vi "FunctionalTest.vi"() -> ()   [LabVIEW 2018]
panel:
  out "TEST RESULT":bool
  out "Functional Test\nErrors":bool[](array[boolean])
  out "SAT":u32[](array[numeric])
  out "HUE":dbl[](array[numeric])
  in  "Port selection":refnum<visa-resource-name>="ASRL27::INSTR"
  out "Status":string
  out "LED 20":bool
  out "LED 19":bool
  out "LED 18":bool
  out "LED 17":bool
  out "LED 16":bool
  out "LED 15":bool
  out "LED 14":bool
  out "LED 13":bool
  out "LED 12":bool
  out "LED 11":bool
  out "LED 10":bool
  out "LED 9":bool
  out "LED 8":bool
  out "LED 7":bool
  out "LED 6":bool
  out "LED 5":bool
  out "LED 4":bool
  out "LED 3":bool
  out "LED 2":bool
  out "LED":bool
  out "INTENSITY":u32[](array[numeric])
  out "BLUE":u8[](array[numeric])
  out "GREEN":u8[](array[numeric])
  out "RED":u8[](array[numeric])
  in  "CAPTURE\n& READ":bool
  in  "stop":bool
  # "Fiber"
  # "1"
  # "2"
  # "3"
  # "4"
  # "5"
  # "6"
  # "7"
  # "8"
  # "9"
  # "10"
  # "11"
  # "12"
  # "13"
  # "14"
  # "15"
  # "16"
  # "17"
  # "18"
  # "19"
  # "20"
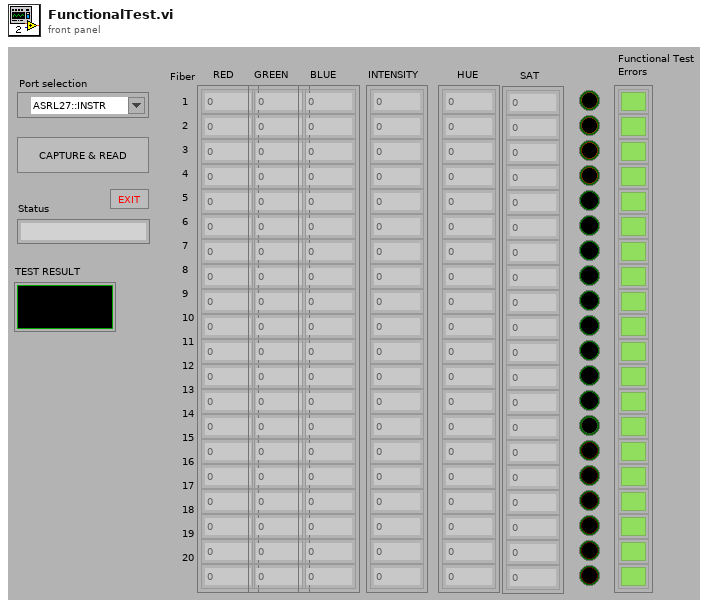
[diagram p1: front panel]
types:
  T1 = enum16{"open", "open or create", "create or replace", "create", "open (read only)"}
  T2 = enum16{"open", "replace", "create", "open or create", "replace or create", "replace or create with confirmation"}
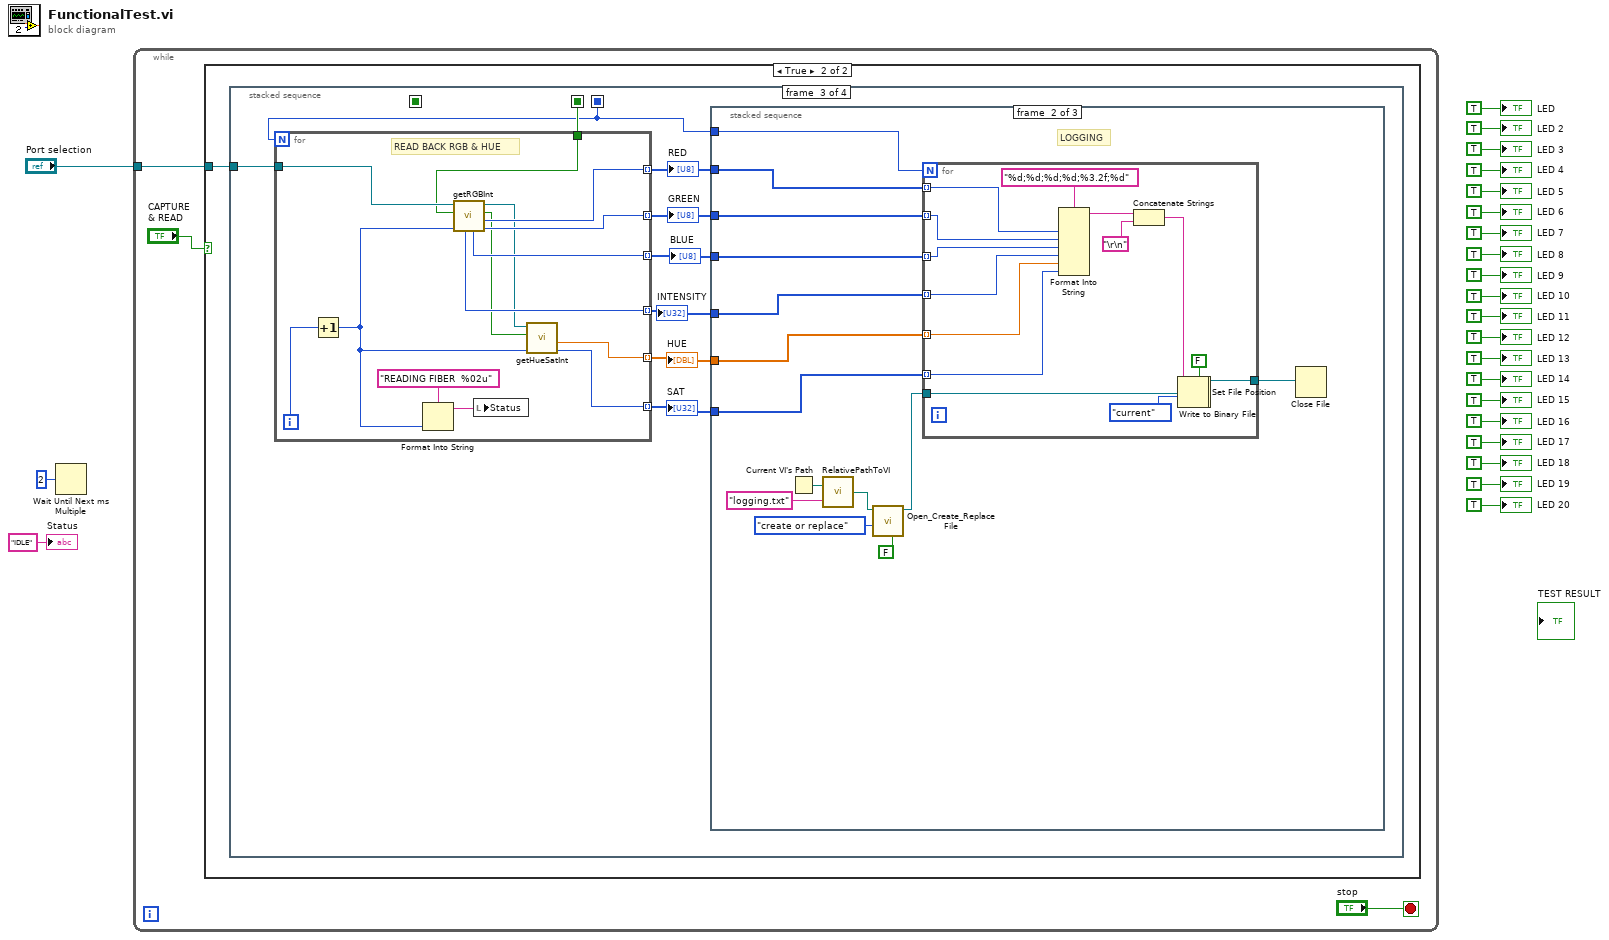
[diagram p0: block diagram]
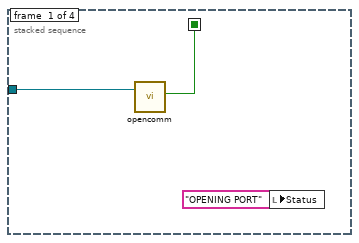
[diagram p3: hidden frame]
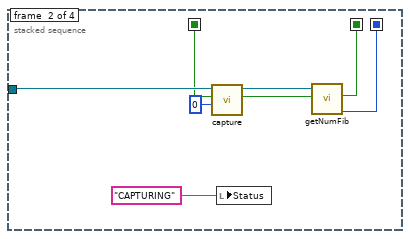
[diagram p4: hidden frame]
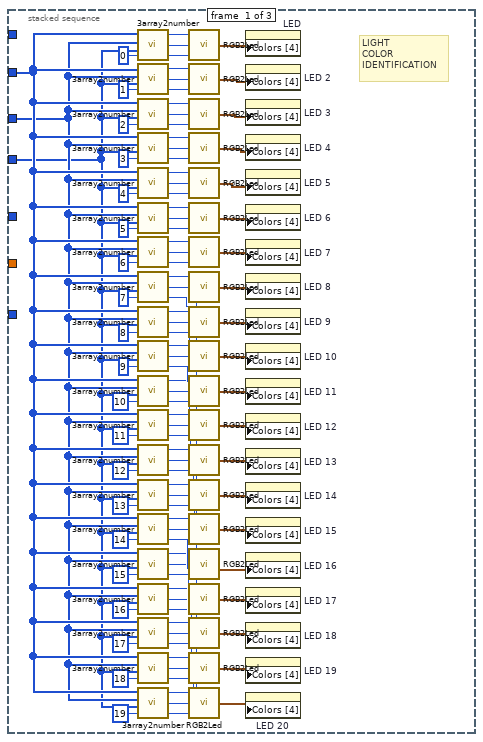
[diagram p5: hidden frame]
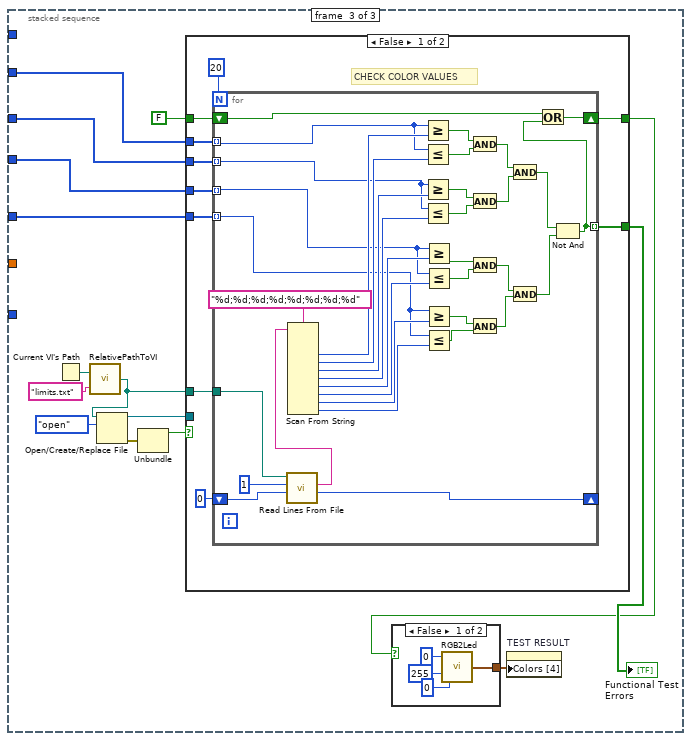
[diagram p6: hidden frame]
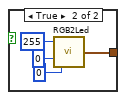
[diagram p7: hidden frame]
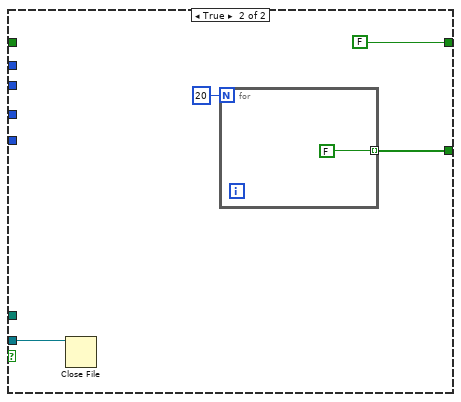
[diagram p8: hidden frame]
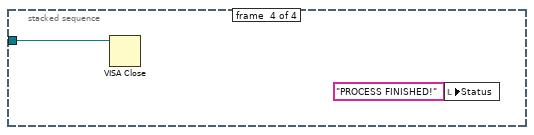
[diagram p9: hidden frame]
diagram:
  n1 = Wait Until Next ms Multiple(millisecond multiple=u32 2) -> ()  [unwired: 1 out]
  n2 = while {
    tunnel: "Port selection" -> [w25]
    stop <- "stop" stop-if-true
    n3 = case shown="True" "CAPTURE\n& READ" {
      tunnel: w25 -> [_ w27]
      frame False {
      }
      frame True {
        n4 = stacked-sequence {
          seq-local: [_ w33 _ _] -> [_ _ w39 _]
          seq-local: [w28 _ _ _] -> [_ w32 _ _]
          seq-local: [_ w31 _ _] -> [_ _ w40 _]
          tunnel: w27 -> [w29 w37 w47 w269]
          frame #0 {
            n5 = call "opencomm.vi"("VISA resource name"=w29) -> ("Error"=w28:bool)  [unwired: 3 in, 1 out]
            n6 = local write "Status"("OPENING PORT" ("Status")) -> ()
          }
          frame #1 {
            n7 = call "capture.vi"("Capture Range (0, auto)"=0 ("Capture Mode (default auto)"), "isPWM (no)"=w32, "VISA resource name"=w37) -> ("Error"=w34:bool, "dup VISA resource name"=w35:refnum<visa-resource-name>)  [unwired: 3 in]
            n8 = local write "Status"("CAPTURING" ("Status")) -> ()
            n9 = call "getNumFib.vi"("Error"=w34, "VISA resource name"=w35) -> ("Fiber Count"=w33:i32, "Error"=w31:bool)  [unwired: 3 in, 1 out]
          }
          frame #2 {
            n10 = for {
              N: w39 -> [_]
              tunnel: w47 -> [w267]
              tunnel: [w262] -> w45 mode=indexing
              tunnel: [w261] -> w44 mode=indexing
              tunnel: [w260] -> w43 mode=indexing
              tunnel: [w259] -> w46 mode=indexing
              tunnel: [w258] -> w42 mode=indexing
              tunnel: [w257] -> w41 mode=indexing
              tunnel: w40 -> [w256]
              i -> [w263]
              # "READ BACK RGB & HUE"
              n11 = Increment(x=w263) -> (x+1=w264:i32)
              n12 = Format Into String(format string="READING FIBER  %02u" ("Status"), w264) -> (resulting string=w265:string)  [unwired: 2 in, 1 out]
              n13 = call "getRGBInt.vi"("Fiber Num"=w264, "Error"=w256, "VISA resource name"=w267) -> ("Green"=w261:u8, "Red"=w262:u8, "Error"=w254:bool, "dup VISA resource name"=w255:refnum<visa-resource-name>, "Blue"=w260:u8, "Intensity"=w259:u32)  [unwired: 3 in]
              n14 = local write "Status"(w265) -> ()
              n15 = call "getHueSatInt.vi"("Fiber Num"=w264, "Error"=w254, "VISA resource name"=w255) -> ("Saturation"=w257:u32, "Hue"=w258:dbl)  [unwired: 2 in, 3 out]
            }
            "RED" <- w45
            "BLUE" <- w43
            "GREEN" <- w44
            "INTENSITY" <- w46
            "HUE" <- w42
            "SAT" <- w41
            n16 = stacked-sequence {
              tunnel: w45 -> [w70 w161 w194]
              tunnel: w44 -> [w69 w160 w193]
              tunnel: w43 -> [w68 w159 w192]
              tunnel: w46 -> [_ w158 w191]
              tunnel: w42 -> [_ w157 _]
              tunnel: w41 -> [_ w156 _]
              tunnel: w39 -> [_ w151 _]
              frame #0 {
                # "LIGHT\nCOLOR\nIDENTIFICATION"
                n17 = call "3array2number.vi"("Index"=0, "Array3"=w68, "Array 2"=w69, "Array1"=w70) -> ("VAL3"=w147:u8, "VAL2"=w149:u8, "VAL1"=w150:u8)
                n18 = call "3array2number.vi"("Index"=1, "Array3"=w68, "Array 2"=w69, "Array1"=w70) -> ("VAL3"=w144:u8, "VAL2"=w145:u8, "VAL1"=w146:u8)
                n19 = call "3array2number.vi"("Index"=2, "Array3"=w68, "Array 2"=w69, "Array1"=w70) -> ("VAL3"=w141:u8, "VAL2"=w142:u8, "VAL1"=w143:u8)
                n20 = call "3array2number.vi"("Index"=3, "Array3"=w68, "Array 2"=w69, "Array1"=w70) -> ("VAL3"=w138:u8, "VAL2"=w139:u8, "VAL1"=w140:u8)
                n21 = call "3array2number.vi"("Index"=4, "Array3"=w68, "Array 2"=w69, "Array1"=w70) -> ("VAL3"=w135:u8, "VAL2"=w136:u8, "VAL1"=w137:u8)
                n22 = call "3array2number.vi"("Index"=5, "Array3"=w68, "Array 2"=w69, "Array1"=w70) -> ("VAL3"=w132:u8, "VAL2"=w133:u8, "VAL1"=w134:u8)
                n23 = call "3array2number.vi"("Index"=6, "Array3"=w68, "Array 2"=w69, "Array1"=w70) -> ("VAL3"=w129:u8, "VAL2"=w130:u8, "VAL1"=w131:u8)
                n24 = call "3array2number.vi"("Index"=7, "Array3"=w68, "Array 2"=w69, "Array1"=w70) -> ("VAL3"=w126:u8, "VAL2"=w127:u8, "VAL1"=w128:u8)
                n25 = call "3array2number.vi"("Index"=8, "Array3"=w68, "Array 2"=w69, "Array1"=w70) -> ("VAL3"=w123:u8, "VAL2"=w124:u8, "VAL1"=w125:u8)
                n26 = call "3array2number.vi"("Index"=9, "Array3"=w68, "Array 2"=w69, "Array1"=w70) -> ("VAL3"=w120:u8, "VAL2"=w121:u8, "VAL1"=w122:u8)
                n27 = call "3array2number.vi"("Index"=10, "Array3"=w68, "Array 2"=w69, "Array1"=w70) -> ("VAL3"=w117:u8, "VAL2"=w118:u8, "VAL1"=w119:u8)
                n28 = call "3array2number.vi"("Index"=11, "Array3"=w68, "Array 2"=w69, "Array1"=w70) -> ("VAL3"=w114:u8, "VAL2"=w115:u8, "VAL1"=w116:u8)
                n29 = call "3array2number.vi"("Index"=12, "Array3"=w68, "Array 2"=w69, "Array1"=w70) -> ("VAL3"=w111:u8, "VAL2"=w112:u8, "VAL1"=w113:u8)
                n30 = call "3array2number.vi"("Index"=13, "Array3"=w68, "Array 2"=w69, "Array1"=w70) -> ("VAL3"=w108:u8, "VAL2"=w109:u8, "VAL1"=w110:u8)
                n31 = call "3array2number.vi"("Index"=14, "Array3"=w68, "Array 2"=w69, "Array1"=w70) -> ("VAL3"=w105:u8, "VAL2"=w106:u8, "VAL1"=w107:u8)
                n32 = call "3array2number.vi"("Index"=15, "Array3"=w68, "Array 2"=w69, "Array1"=w70) -> ("VAL3"=w98:u8, "VAL2"=w99:u8, "VAL1"=w100:u8)
                n33 = call "3array2number.vi"("Index"=16, "Array3"=w68, "Array 2"=w69, "Array1"=w70) -> ("VAL3"=w95:u8, "VAL2"=w96:u8, "VAL1"=w97:u8)
                n34 = call "3array2number.vi"("Index"=17, "Array3"=w68, "Array 2"=w69, "Array1"=w70) -> ("VAL3"=w92:u8, "VAL2"=w93:u8, "VAL1"=w94:u8)
                n35 = call "3array2number.vi"("Index"=18, "Array3"=w68, "Array 2"=w69, "Array1"=w70) -> ("VAL3"=w89:u8, "VAL2"=w90:u8, "VAL1"=w91:u8)
                n36 = call "3array2number.vi"("Index"=19, "Array3"=w68, "Array 2"=w69, "Array1"=w70) -> ("VAL3"=w86:u8, "VAL2"=w87:u8, "VAL1"=w88:u8)
                n37 = call "RGB2Led.vi"("B"=w147, "G"=w149, "R"=w150) -> ("Colors [4]"=w148:cluster{u32, u32}[])
                n38 = call "RGB2Led.vi"("B"=w144, "G"=w145, "R"=w146) -> ("Colors [4]"=w104:cluster{u32, u32}[])
                n39 = call "RGB2Led.vi"("B"=w141, "G"=w142, "R"=w143) -> ("Colors [4]"=w103:cluster{u32, u32}[])
                n40 = call "RGB2Led.vi"("B"=w138, "G"=w139, "R"=w140) -> ("Colors [4]"=w102:cluster{u32, u32}[])
                n41 = call "RGB2Led.vi"("B"=w135, "G"=w136, "R"=w137) -> ("Colors [4]"=w101:cluster{u32, u32}[])
                n42 = call "RGB2Led.vi"("B"=w132, "G"=w133, "R"=w134) -> ("Colors [4]"=w85:cluster{u32, u32}[])
                n43 = call "RGB2Led.vi"("B"=w129, "G"=w130, "R"=w131) -> ("Colors [4]"=w84:cluster{u32, u32}[])
                n44 = call "RGB2Led.vi"("B"=w126, "G"=w127, "R"=w128) -> ("Colors [4]"=w83:cluster{u32, u32}[])
                n45 = call "RGB2Led.vi"("B"=w123, "G"=w124, "R"=w125) -> ("Colors [4]"=w82:cluster{u32, u32}[])
                n46 = call "RGB2Led.vi"("B"=w120, "G"=w121, "R"=w122) -> ("Colors [4]"=w81:cluster{u32, u32}[])
                n47 = call "RGB2Led.vi"("B"=w117, "G"=w118, "R"=w119) -> ("Colors [4]"=w80:cluster{u32, u32}[])
                n48 = call "RGB2Led.vi"("B"=w114, "G"=w115, "R"=w116) -> ("Colors [4]"=w79:cluster{u32, u32}[])
                n49 = call "RGB2Led.vi"("B"=w111, "G"=w112, "R"=w113) -> ("Colors [4]"=w78:cluster{u32, u32}[])
                n50 = call "RGB2Led.vi"("B"=w108, "G"=w109, "R"=w110) -> ("Colors [4]"=w77:cluster{u32, u32}[])
                n51 = call "RGB2Led.vi"("B"=w105, "G"=w106, "R"=w107) -> ("Colors [4]"=w76:cluster{u32, u32}[])
                n52 = call "RGB2Led.vi"("B"=w98, "G"=w99, "R"=w100) -> ("Colors [4]"=w75:cluster{u32, u32}[])
                n53 = call "RGB2Led.vi"("B"=w95, "G"=w96, "R"=w97) -> ("Colors [4]"=w74:cluster{u32, u32}[])
                n54 = call "RGB2Led.vi"("B"=w92, "G"=w93, "R"=w94) -> ("Colors [4]"=w73:cluster{u32, u32}[])
                n55 = call "RGB2Led.vi"("B"=w89, "G"=w90, "R"=w91) -> ("Colors [4]"=w72:cluster{u32, u32}[])
                n56 = call "RGB2Led.vi"("B"=w86, "G"=w87, "R"=w88) -> ("Colors [4]"=w71:cluster{u32, u32}[])
                n57 = property on="LED" class="Bool (strict)"("Colors [4]"=w148) -> ()  [unwired: 2 in, 2 out]
                n58 = property on="LED 2" class="Bool (strict)"("Colors [4]"=w104) -> ()  [unwired: 2 in, 2 out]
                n59 = property on="LED 3" class="Bool (strict)"("Colors [4]"=w103) -> ()  [unwired: 2 in, 2 out]
                n60 = property on="LED 4" class="Bool (strict)"("Colors [4]"=w102) -> ()  [unwired: 2 in, 2 out]
                n61 = property on="LED 5" class="Bool (strict)"("Colors [4]"=w101) -> ()  [unwired: 2 in, 2 out]
                n62 = property on="LED 6" class="Bool (strict)"("Colors [4]"=w85) -> ()  [unwired: 2 in, 2 out]
                n63 = property on="LED 7" class="Bool (strict)"("Colors [4]"=w84) -> ()  [unwired: 2 in, 2 out]
                n64 = property on="LED 8" class="Bool (strict)"("Colors [4]"=w83) -> ()  [unwired: 2 in, 2 out]
                n65 = property on="LED 9" class="Bool (strict)"("Colors [4]"=w82) -> ()  [unwired: 2 in, 2 out]
                n66 = property on="LED 10" class="Bool (strict)"("Colors [4]"=w81) -> ()  [unwired: 2 in, 2 out]
                n67 = property on="LED 11" class="Bool (strict)"("Colors [4]"=w80) -> ()  [unwired: 2 in, 2 out]
                n68 = property on="LED 12" class="Bool (strict)"("Colors [4]"=w79) -> ()  [unwired: 2 in, 2 out]
                n69 = property on="LED 13" class="Bool (strict)"("Colors [4]"=w78) -> ()  [unwired: 2 in, 2 out]
                n70 = property on="LED 14" class="Bool (strict)"("Colors [4]"=w77) -> ()  [unwired: 2 in, 2 out]
                n71 = property on="LED 15" class="Bool (strict)"("Colors [4]"=w76) -> ()  [unwired: 2 in, 2 out]
                n72 = property on="LED 16" class="Bool (strict)"("Colors [4]"=w75) -> ()  [unwired: 2 in, 2 out]
                n73 = property on="LED 17" class="Bool (strict)"("Colors [4]"=w74) -> ()  [unwired: 2 in, 2 out]
                n74 = property on="LED 18" class="Bool (strict)"("Colors [4]"=w73) -> ()  [unwired: 2 in, 2 out]
                n75 = property on="LED 19" class="Bool (strict)"("Colors [4]"=w72) -> ()  [unwired: 2 in, 2 out]
                n76 = property on="LED 20" class="Bool (strict)"("Colors [4]"=w71) -> ()  [unwired: 2 in, 2 out]
              }
              frame #1 {
                # "LOGGING"
                n77 = Current VI's Path() -> (path=w154:path)
                n78 = call "RelativePathToVI.vi"("Relative Path to VI"="logging.txt", "VI path"=w154) -> ("Absoulte path"=w152:path)
                n79 = call <vilib>:"Open_Create_Replace File.vi"("advisory dialog? (display:T)"=FALSE, "function (open:0)"=T1."create or replace", "file path"=w152) -> ("refnum"=w163:refnum<file>)  [unwired: 5 in, 3 out]
                n80 = for {
                  N: w151 -> [_]
                  tunnel: w163 -> [w180]
                  tunnel: [w178] -> w162
                  tunnel: w161 -> [w172] mode=indexing
                  tunnel: w160 -> [w171] mode=indexing
                  tunnel: w159 -> [w170] mode=indexing
                  tunnel: w158 -> [w169] mode=indexing
                  tunnel: w157 -> [w168] mode=indexing
                  tunnel: w156 -> [w167] mode=indexing
                  n81 = Format Into String(format string="%d;%d;%d;%d;%3.2f;%d", w172, w171, w170, w169, w168, w167) -> (resulting string=w166:string)  [unwired: 2 in, 1 out]
                  n82 = Concatenate Strings(w166, "\r\n") -> (w177:string)
                  n83 = Set File Position(refnum=w180, from (0:start)=enum16{"start", "end", "current"}."current" ("pos mode (0:2)")) -> (refnum out=w176:refnum<file>, error out=w175:errorcluster)  [unwired: 2 in]
                  n84 = Write to Binary File(file (use dialog)=w176, data=w177, error in=w175, 5:FALSE ("prepend array or string size? (T)")) -> (refnum out=w178:refnum<file>)  [unwired: 2 in, 2 out]
                }
                n85 = Close File(refnum=w162) -> ()  [unwired: 1 in, 2 out]
              }
              frame #2 {
                n86 = Current VI's Path() -> (path=w183:path)
                n87 = call "RelativePathToVI.vi"("Relative Path to VI"="limits.txt", "VI path"=w183) -> ("Absoulte path"=w181:path)
                n88 = Open/Create/Replace File(file path (use dialog)=w181, operation (0:open)=T2."open") -> (refnum out=w189:refnum<file>, error out=w188:errorcluster)  [unwired: 4 in, 1 out]
                n89 = Unbundle(w188) -> ("status"=w187:bool)  [unwired: 2 out]
                n90 = case shown="False" w187 {
                  tunnel: [w211 w251] -> w195
                  tunnel: w194 -> [w210 _]
                  tunnel: w193 -> [w209 _]
                  tunnel: w192 -> [w208 _]
                  tunnel: w191 -> [w207 _]
                  tunnel: w189 -> [_ w252]
                  tunnel: [w205 FALSE] -> w185
                  tunnel: FALSE ("LED 18") -> [w206 _]
                  tunnel: w181 -> [w204 _]
                  frame False {
                    # "CHECK COLOR VALUES"
                    n91 = for {
                      N: 20 -> [_]
                      tunnel: w210 -> [w217] mode=indexing
                      tunnel: w209 -> [w216] mode=indexing
                      tunnel: w208 -> [w215] mode=indexing
                      tunnel: w207 -> [w214] mode=indexing
                      shift-right: [w248] -> _
                      shift-left: 0 ("mark after read (chars.)") -> [w247]
                      tunnel: [w219] -> w211 mode=indexing
                      shift-right: [w220] -> w205
                      shift-left: w206 -> [w221]
                      tunnel: w204 -> [w218]
                      n92 = call <vilib>:"Read Lines From File.vi"("file path (dialog if empty)"=w218, "number of lines (all:-1)"=1, "start of read offset (chars.:0)"=w247) -> ("line string"=w244:string, "mark after read (chars.)"=w248:i32)  [unwired: 3 in, 2 out]
                      n93 = Scan From String(format string="%d;%d;%d;%d;%d;%d;%d;%d" ("Format String"), input string=w244) -> (output 1=w243:i32, output 2=w242:i32, output 3=w241:i32, output 4=w240:i32, output 5=w239:i32, output 6=w238:i32, output 7=w237:i32, output 8=w236:i32)  [unwired: 10 in, 3 out]
                      n94 = Greater Or Equal?(x=w217, y=w243) -> (x >= y?=w229:bool)
                      n95 = Less Or Equal?(x=w217, y=w242) -> (x <= y?=w228:bool)
                      n96 = Greater Or Equal?(x=w216, y=w241) -> (x >= y?=w227:bool)
                      n97 = Less Or Equal?(x=w216, y=w240) -> (x <= y?=w226:bool)
                      n98 = Greater Or Equal?(x=w215, y=w239) -> (x >= y?=w225:bool)
                      n99 = Less Or Equal?(x=w215, y=w238) -> (x <= y?=w224:bool)
                      n100 = Greater Or Equal?(x=w214, y=w237) -> (x >= y?=w223:bool)
                      n101 = Less Or Equal?(x=w214, y=w236) -> (x <= y?=w222:bool)
                      n102 = And(x=w229, y=w228) -> (x .and. y?=w233:bool)
                      n103 = And(x=w227, y=w226) -> (x .and. y?=w232:bool)
                      n104 = And(x=w225, y=w224) -> (x .and. y?=w231:bool)
                      n105 = And(x=w223, y=w222) -> (x .and. y?=w230:bool)
                      n106 = And(x=w233, y=w232) -> (x .and. y?=w235:bool)
                      n107 = And(x=w231, y=w230) -> (x .and. y?=w234:bool)
                      n108 = Not And(1:w234, 2:w235) -> (0:w219:bool)
                      n109 = Or(x=w221, y=w219) -> (x .or. y?=w220:bool)
                    }
                  }
                  frame True {
                    n110 = Close File(refnum=w252) -> ()  [unwired: 1 in, 2 out]
                    n111 = for {
                      N: 20 -> [_]
                      tunnel: [FALSE] -> w251 mode=indexing
                    }
                  }
                }
                "Functional Test\nErrors" <- w195
                n112 = case shown="False" w185 {
                  tunnel: [w196 w200] -> w184
                  frame False {
                    n113 = call "RGB2Led.vi"("B"=u32 0, "G"=u32 255, "R"=u32 0) -> ("Colors [4]"=w196:cluster{u32, u32}[])
                  }
                  frame True {
                    n114 = call "RGB2Led.vi"("B"=u32 0, "G"=u32 0, "R"=u32 255) -> ("Colors [4]"=w200:cluster{u32, u32}[])
                  }
                }
                n115 = property on="TEST RESULT" class="Bool (strict)"("Colors [4]"=w184) -> ()  [unwired: 2 in, 2 out]
              }
            }
          }
          frame #3 {
            n116 = VISA Close(VISA resource name=w269) -> ()  [unwired: 1 in, 1 out]
            n117 = local write "Status"("PROCESS FINISHED!" ("Status")) -> ()
          }
        }
      }
    }
  }
  "LED" <- TRUE ("LED")
  "LED 2" <- TRUE ("LED 2")
  "LED 3" <- TRUE ("LED 3")
  "LED 4" <- TRUE ("LED 4")
  "LED 5" <- TRUE ("LED 5")
  "LED 6" <- TRUE ("LED 6")
  "LED 11" <- TRUE ("LED 11")
  "LED 10" <- TRUE ("LED 10")
  "LED 9" <- TRUE ("LED 9")
  "LED 8" <- TRUE ("LED 8")
  "LED 7" <- TRUE ("LED 7")
  "LED 16" <- TRUE ("LED 16")
  "LED 15" <- TRUE ("LED 15")
  "LED 14" <- TRUE ("LED 14")
  "LED 13" <- TRUE ("LED 13")
  "LED 12" <- TRUE ("LED 12")
  "LED 20" <- TRUE ("LED 20")
  "LED 19" <- TRUE ("LED 19")
  "LED 18" <- TRUE ("LED 18")
  "LED 17" <- TRUE ("LED 17")
  "Status" <- "IDLE" ("Status")
